vi "Empty_Check.vi"(8 "error in (no error)":errorcluster, 11 "Boolean":bool) -> (0 "error out":errorcluster)   [LabVIEW 2017]
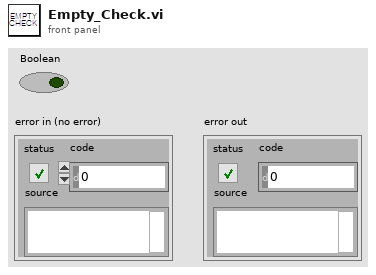
[diagram p1: front panel]
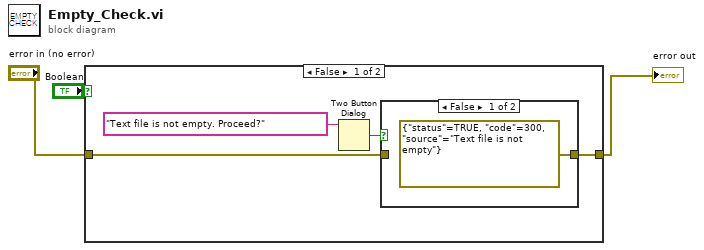
[diagram p0: block diagram]
diagram:
  n1 = case shown="False" "Boolean" {
    tunnel: "error in (no error)" -> [w5 w10]
    tunnel: [w4 w10] -> w3
    frame False {
      n2 = Two Button Dialog(message="Text file is not empty. Proceed?") -> (T button?=w6:bool)  [unwired: 2 in]
      n3 = case shown="False" w6 {
        tunnel: w5 -> [_ w9]
        tunnel: [errorcluster {"status"=TRUE, "code"=300, "source"="Text file is not empty"} ("error constant") w9] -> w4
        frame False {
        }
        frame True {
        }
      }
    }
    frame True {
    }
  }
  "error out" <- w3
